vi "Get Performance.vi"(11 "Framework Status in":refnum<class "Framework Status.lvclass">) -> (2 "Framework Performance":refnum<class "Framework Performance.lvclass">, 3 "Framework Status out":refnum<class "Framework Status.lvclass">)   [LabVIEW 2017, in "Data Sharing Framework Core.lvlib" / "Data Sharing Framework Engine.lvlib" / "Framework Status.lvclass"]
uses:
  Framework Status.lvclass
  Framework Performance/Framework Performance.lvclass
  Framework Status.lvclass/Framework Status.ctl
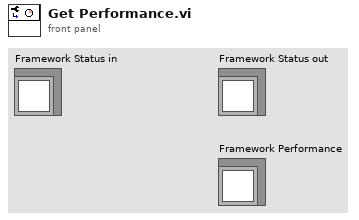
[diagram p1: front panel]
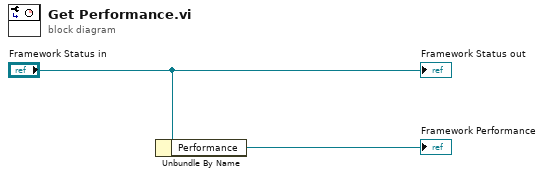
[diagram p0: block diagram]
diagram:
  n1 = Unbundle By Name("Framework Status in") -> ("Performance"=→"Framework Performance":refnum<class "Framework Performance.lvclass">)
  "Framework Status out" <- "Framework Status in"
